vi "Calc Dist to ConstV.vi"(10 "Limits":T1={"Velocity (fps)"=10.0, "Acceleration (fps^2)"=10.0, "Jerk (fps^3)"=100.0}, 11 "V endpoint (fps)":dbl) -> (0 "dist of high Jerk":dbl, 1 "dist of baseline Jerk":dbl, 2 "Time to const V":dbl, 3 "distance (ft)":dbl)   [LabVIEW 2020]
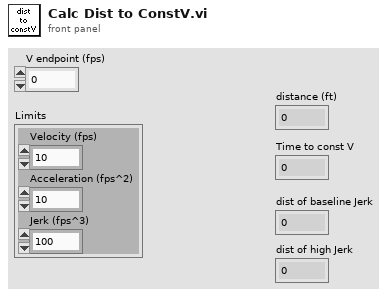
[diagram p1: front panel]
types:
  T1 = cluster{"Velocity (fps)":dbl, "Acceleration (fps^2)":dbl, "Jerk (fps^3)":dbl}
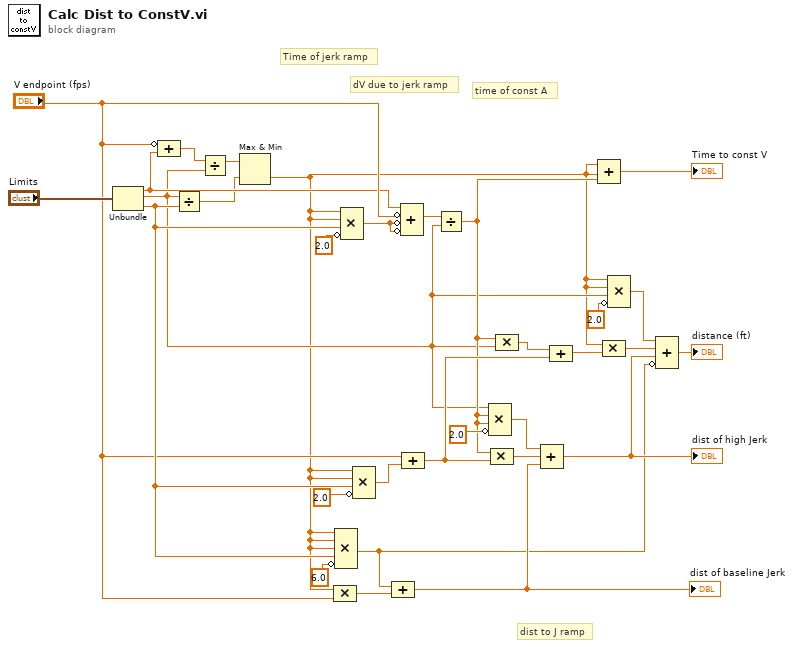
[diagram p0: block diagram]
diagram:
  # "dist to J ramp"
  # "time of const A"
  # "dV due to jerk ramp"
  # "Time of jerk ramp"
  n1 = Unbundle("Limits") -> ("Velocity (fps)"=w6:dbl, "Acceleration (fps^2)"=w4:dbl, "Jerk (fps^3)"=w16:dbl)
  n2 = Compound Arithmetic op=ADD(invert "V endpoint (fps)", w6) -> (w5:dbl)
  n3 = Divide(x=w4, y=w16) -> (x/y=w2:dbl)
  n4 = Divide(x=w5, y=w4) -> (x/y=w3:dbl)
  n5 = Max & Min(x=w3, y=w2) -> (min(x,y)=w1:dbl)  [unwired: 1 out]
  n6 = Compound Arithmetic op=MULTIPLY(w1, "V endpoint (fps)") -> (w24:dbl)
  n7 = Compound Arithmetic op=MULTIPLY(w1, w1, w1, w16, invert 6.0) -> (w11:dbl)
  n8 = Compound Arithmetic op=MULTIPLY(w1, w1, w16, invert 2.0) -> (w25:dbl)
  n9 = Compound Arithmetic op=MULTIPLY(w1, w1, w16, invert 2.0) -> (w10:dbl)
  n10 = Compound Arithmetic op=ADD(w11, w24) -> (w22:dbl)
  "dist of baseline Jerk" <- w22
  n11 = Compound Arithmetic op=ADD(w6, invert "V endpoint (fps)", invert w25, invert w25) -> (w29:dbl)
  n12 = Compound Arithmetic op=ADD("V endpoint (fps)", w10) -> (w15:dbl)
  n13 = Divide(x=w29, y=w4) -> (x/y=w14:dbl)
  n14 = Compound Arithmetic op=MULTIPLY(w4, w14, w14, invert 2.0) -> (w20:dbl)
  n15 = Compound Arithmetic op=MULTIPLY(w14, w15) -> (w21:dbl)
  n16 = Compound Arithmetic op=MULTIPLY(w14, w4) -> (w13:dbl)
  n17 = Compound Arithmetic op=ADD(w20, w21, w22) -> (w19:dbl)
  "dist of high Jerk" <- w19
  n18 = Compound Arithmetic op=ADD(w13, w15) -> (w12:dbl)
  n19 = Compound Arithmetic op=ADD(w1, w1, w14) -> (→"Time to const V":dbl)
  n20 = Compound Arithmetic op=MULTIPLY(w1, w12) -> (w18:dbl)
  n21 = Compound Arithmetic op=MULTIPLY(w1, w1, w4, invert 2.0) -> (w8:dbl)
  n22 = Compound Arithmetic op=ADD(w8, w18, w19, invert w11) -> (→"distance (ft)":dbl)
